vi "Create voltage list.vi"(6 "No. of measurement points":dbl, 7 "Sweep Direction":u16, 9 "No. of data point averages":dbl, 10 "Maximum voltage (V)":dbl, 11 "Minimum voltage (V)":dbl) -> (2 "Voltages":dbl[](array[numeric]), 3 "Voltage list for measurement":dbl[](array[numeric]))   [LabVIEW 2011]
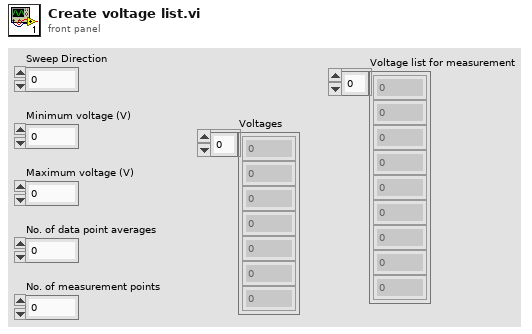
[diagram p1: front panel]
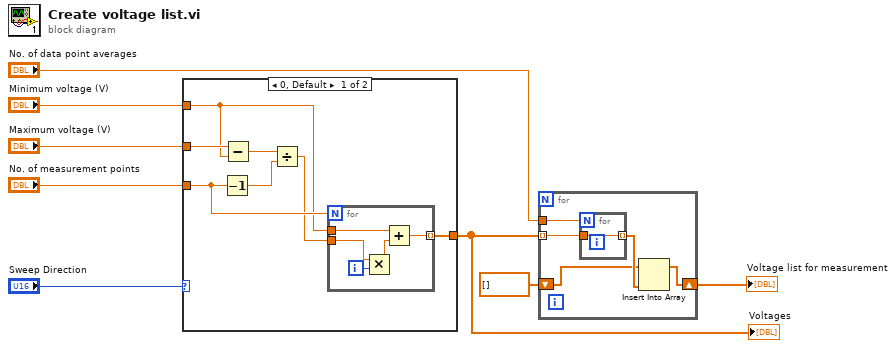
[diagram p0: block diagram]
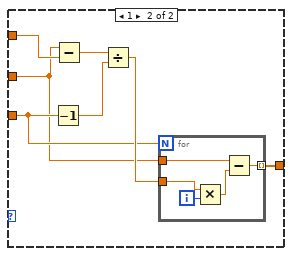
[diagram p2: hidden frame]
diagram:
  n1 = case shown="0, Default" "Sweep Direction" {
    tunnel: "No. of measurement points" -> [w14 w22]
    tunnel: "Maximum voltage (V)" -> [w12 w21]
    tunnel: "Minimum voltage (V)" -> [w11 w23]
    tunnel: [w9 w24] -> w1
    frame 0, Default {
      n2 = Decrement(x=w14) -> (x-1=w15:dbl)
      n3 = Subtract(x=w12, y=w11) -> (x-y=w10:dbl)
      n4 = Divide(x=w10, y=w15) -> (x/y=w13:dbl)
      n5 = for {
        N: w14 -> [_]
        tunnel: w11 -> [w20]
        tunnel: w13 -> [w17]
        tunnel: [w19] -> w9 mode=indexing
        i -> [w18]
        n6 = Multiply(x=w17, y=w18) -> (x*y=w16:dbl)
        n7 = Add(x=w20, y=w16) -> (x+y=w19:dbl)
      }
    }
    frame 1 {
      n8 = Decrement(x=w22) -> (x-1=w27:dbl)
      n9 = Subtract(x=w21, y=w23) -> (x-y=w25:dbl)
      n10 = Divide(x=w25, y=w27) -> (x/y=w26:dbl)
      n11 = for {
        N: w22 -> [_]
        tunnel: w26 -> [w30]
        tunnel: [w32] -> w24 mode=indexing
        tunnel: w21 -> [w28]
        i -> [w31]
        n12 = Multiply(x=w30, y=w31) -> (x*y=w29:dbl)
        n13 = Subtract(x=w28, y=w29) -> (x-y=w32:dbl)
      }
    }
  }
  "Voltages" <- w1
  n14 = for {
    tunnel: w1 -> [w37] mode=indexing
    shift-right: [w36] -> w3
    shift-left: dbl[] [] -> [w34]
    tunnel: "No. of data point averages" -> [w33]
    n15 = for {
      N: w33 -> [_]
      tunnel: w37 -> [w38]
      tunnel: [w38] -> w35 mode=indexing
    }
    n16 = Insert Into Array(array=w34, new element=w35) -> (w36:dbl[])  [unwired: 1 in]
  }
  "Voltage list for measurement" <- w3
